vi "WriteDataByIdentifier.vi"(5 "LogSuspend":bool, 8 "error in":errorcluster, 9 "DataIn":string="02 02", 10 "DID":string="02 02", 11 "UdsHandleIn":T1={"LogPath"=path "", "LogEnabled"=FALSE, "isOpen"=FALSE, "LogContent"="", "Adapter"="CAN0", "MCanHandle"={"MCanAdapter"=refnum}, "TransmittId"=0, "ReceiveId"=0}) -> (0 "error out":errorcluster, 3 "UdsHandleOut":T1={"LogPath"=path "", "LogEnabled"=FALSE, "isOpen"=FALSE, "LogContent"="", "Adapter"="CAN0", "MCanHandle"={"MCanAdapter"=refnum}, "TransmittId"=0, "ReceiveId"=0})   [LabVIEW 2011, in "Konvolucio MUDS150628.lvlib"]
uses:
  <instrlib>/Konvolucio MUDS150628/Konvolucio MUDS150628.lvlib
  <instrlib>/Konvolucio MUDS150628/Types/UdsHandleType.ctl
  <instrlib>/Konvolucio MCAN120803/Types/MCanHandleType.ctl
  C:/Program Files/National Instruments/LabVIEW 2011/instr.lib/Konvolucio MCAN120803/Private/Konvolucio.MCAN120803.dll
  Konvolucio MCAN120803/Private/Konvolucio.MCAN120803.dll
  <instrlib>/Konvolucio MCAN120803/Konvolucio MCAN120803.lvlib
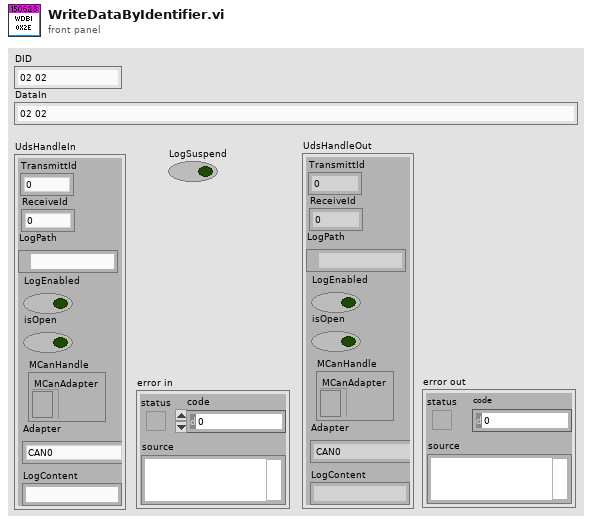
[diagram p1: front panel]
types:
  T1 = typedef "Konvolucio MUDS150628.lvlib/UdsHandleType.ctl" = cluster{"LogPath":path, "LogEnabled":bool, "isOpen":bool, "LogContent":string, "Adapter":string, "MCanHandle":T2, "TransmittId":u32, "ReceiveId":u32}
  T2 = typedef "Konvolucio MCAN120803.lvlib/MCanHandleType.ctl" = cluster{"MCanAdapter":refnum<k24>}
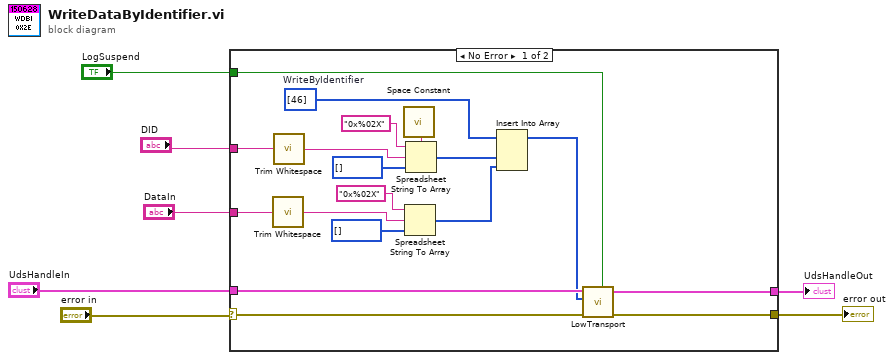
[diagram p0: block diagram]
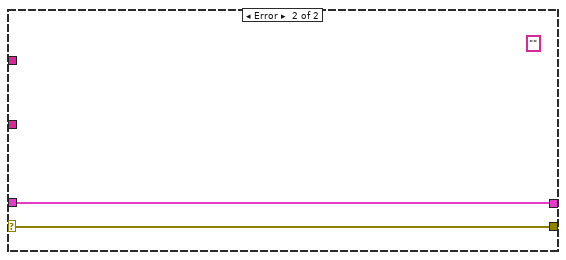
[diagram p2: hidden frame]
diagram:
  n1 = case shown="No Error" "error in" {
    selector: "error in" -> [w24 w27]
    tunnel: "UdsHandleIn" -> [w25 w26]
    tunnel: [w23 w27] -> w5
    tunnel: [w22 w26] -> w4
    tunnel: "LogSuspend" -> [w21 _]
    tunnel: "DID" -> [w13 _]
    tunnel: "DataIn" -> [w10 _]
    frame No Error {
      w20 = u8[] [46]  # WriteByIdentifier
      n2 = call <vilib>:"Trim Whitespace.vi"("string"=w10) -> ("trimmed string"=w11:string)  [unwired: 1 in]
      n3 = call <vilib>:"Trim Whitespace.vi"("string"=w13) -> ("trimmed string"=w19:string)  [unwired: 1 in]
      n4 = call <vilib>:"Space Constant.vi"() -> ("String"=w18:string)
      n5 = Spreadsheet String To Array(format string="0x%02X", spreadsheet string=w11, array type (2D Dbl)=u8[] [] ("Response")) -> (array=w9:u8[])  [unwired: 1 in]
      n6 = Spreadsheet String To Array(delimiter (Tab)=w18, format string="0x%02X", spreadsheet string=w19, array type (2D Dbl)=u8[] [] ("Response")) -> (array=w15:u8[])
      n7 = Insert Into Array(array=w20, new element #1=w15, new element #2=w9) -> (w14:u8[])  [unwired: 1 in]
      n8 = call <instrlib>:"LowTransport.vi"("LogSuspend"=w21, "error in"=w24, "Request"=w14, "HandleIn"=w25) -> ("error out"=w23:errorcluster, "HandleOut"=w22:T1)  [unwired: 5 in, 1 out]
    }
    frame Error {
      (unwired) "" ("trimmed string")
    }
  }
  "error out" <- w5
  "UdsHandleOut" <- w4
